vi "Dashboard Main_1366_768.vi"() -> ()   [LabVIEW 2020]
uses:
  <vilib>/event_ctls.llb/eventvkey.ctl
  <vilib>/Rock Robotics/WPI/Dashboard/WPI_DashboardLogging Global.vi
  <vilib>/Rock Robotics/Network Tables/NT Read Boolean.vi
panel:
  out "Camera Perf":string
  in  "Camera Settings":T1={"Frame Rate"=30, "Compression"=30, "Size"=1, "DB Camera Config"=FALSE} {"Frame Rate" scale=1.0..30.0; "Compression" scale=100.0..-1.0; "Size" items=["640x480", "320x240", "160x120"]}
  in  "TCP":refnum<k5>
  in  "Rec Mode":enum32{"Stop", "Record", "Playback"}(radio)
  out "Robot IP":string
  out "Image Message":string="Timeout in Camera Communications"
  in  "Dashboard Tab":T2(tab)
  in  "Select Auto":string(combo)="Select Autonomous ..."
  out "NT Connection":bool
  out "JS1 Z":dbl(slide) scale=-1.0..1.0 scale format="%#_2e"
  out "JS1 Graph":cluster{"X":dbl, "Y":dbl}[](graph)
  out "JS1 Buttons":T3
  out "JS2 Z":dbl(slide) scale=-1.0..1.0 scale format="%#_2e"
  out "JS2 Graph":cluster{"X":dbl, "Y":dbl}[](graph)
  out "JS2 Buttons":T3
  out "Mode":T4(ring)=enum."Auto Disabled"
  out "Right Camera Perf":cluster{"Bandwidth (Mbps)":dbl, "FPS":dbl}
  out "Middle":bool
  out "Bottom":bool
  out "Game\nPiece":bool
  out "Top":bool
  out "Shelf":bool
  out "Floor":bool
  out "MtT":bool
  out "At Target":bool
  out "Arm Override":bool
  out "Speed Modifer":dbl
  out "Reverse":bool
  out "Current Action":string
  out "ExtendDmd":dbl
  out "LiftDmd":dbl
  in  "DB/String 9":string
  in  "DB/String 8":string
  in  "DB/String 7":string
  in  "DB/String 6":string
  in  "DB/String 5":string
  in  "DB/String 4":string
  in  "DB/String 3":string
  in  "DB/String 2":string
  in  "DB/String 1":string
  in  "DB/String 0":string
  in  "DB/Slider 0":dbl(slide) scale=0.0..5.0
  in  "DB/Slider 1":dbl(slide) scale=0.0..5.0
  in  "DB/Slider 2":dbl(slide) scale=0.0..5.0
  in  "DB/Slider 3":dbl(slide) scale=0.0..5.0
  out "DB/LED 3":bool
  out "DB/LED 2":bool
  out "DB/LED 1":bool
  out "DB/LED 0":bool
  in  "DB/Button 3":bool
  in  "DB/Button 2":bool
  in  "DB/Button 1":bool
  in  "DB/Button 0":bool caption="New Name"
  in  "Test Slider":dbl(slide) scale=0.0..100.0 scale format="%#_3g"
  in  "On/Off":bool caption="Solenoid"
  in  "Test Name":u16(ring) items=["Select the test to run..."]
  in  "Test Tree":string(tree)
  in  "Motor":cluster{"Value":dbl, "Enable":bool} {"Value" scale=-1.0..1.0 scale format="%#_3g"}
  out "Progress":T5 {"Test Progress" scale=0.0..100.0}
  in  "Rev/Fwd":cluster{"Forward":bool, "Reverse":bool}
  in  "Test Ring":u16(ring) items=["Monochrome", "Color"]
  in  "CheckList":i32(listbox)
  out "Tree":string(tree)
  out "Camera Image":T6(plugin-control)
  out "Background":bool
  in  "Camera Name":string(combo)="No Camera Selection"
  # "HW"
  # "Joysticks"
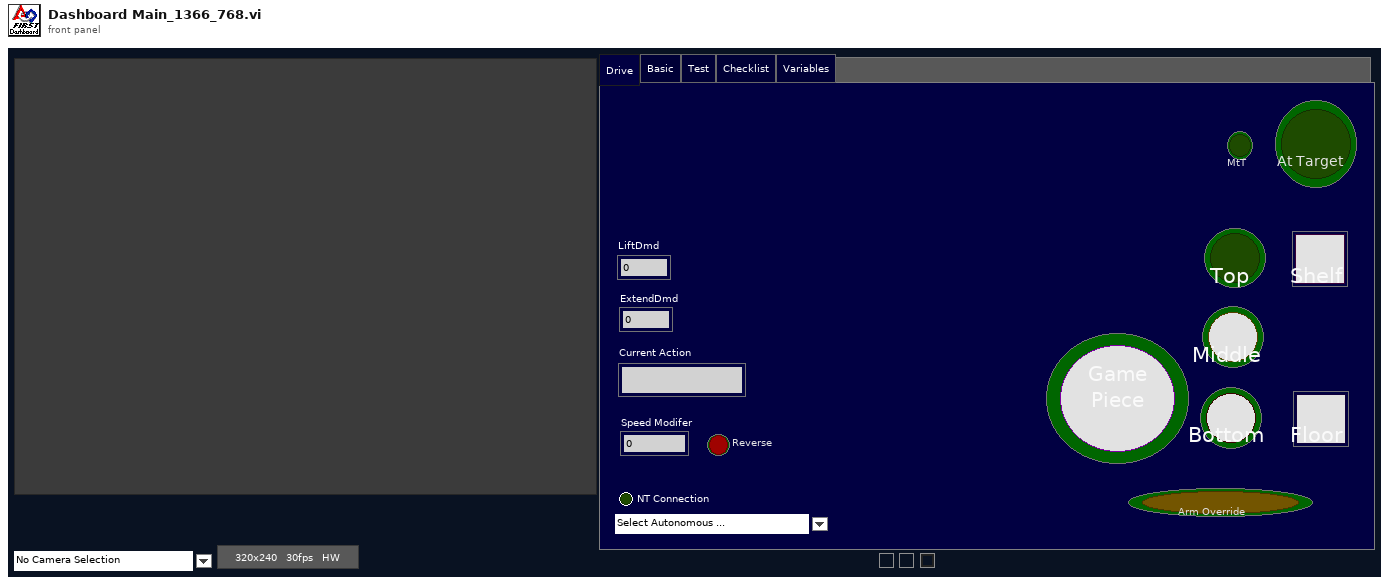
[diagram p1: front panel]
types:
  T1 = cluster{"Frame Rate":i32, "Compression":i32, "Size":u16, "DB Camera Config":bool}
  T2 = enum32{"Drive", "Basic", "Test", "Checklist", "Variables"}
  T3 = cluster{bool, bool, bool, bool, bool, bool, bool, bool, bool, bool, bool, bool}
  T4 = enum8{"Tele-Op Disabled", "Tele-Op Enabled", "Auto Disabled", "Auto Enabled", "Test Disabled", "Test Enabled", "Disconnected", "No Code", "E-Stop"}
  T5 = cluster{"Test Progress":u8, "Test Progress Text":string}
  T6 = typedef "IMAQ Image.ctl" = refnum<image>
  T7 = enum32{"Drive", "Basic", "Custom", "Test", "Checklist", "Variables"}
  T8 = cluster{"Save Path":path, "Interval (s)":dbl, "Keep":i32}
  T9 = enum32{"Drive", "Camera", "Basic", "Custom", "Test", "Commands", "Checklist", "Variables"}
  T10 = typedef "Image Type" = u32
  T11 = cluster{"Error Strings":string, "Disable Counts":cluster{u16, u16}, "Rail Faults":cluster{u16, u16, u16}, "Robot IP":string, "DB Mode":u8, "Event Info":cluster{"Name":string, "Type":u8, "Number":u16, "Replay":u8}}
  T12 = cluster{"Storage":cluster{"Disk Free":u64, "RAM Block":u32, "RAM free":u32}, "CPU Utilization":cluster{"CPU % ISR":sgl, "CPU % Time Crit":sgl, "CPU % Timed Str":sgl, "CPU % High":sgl, "CPU % Above":sgl, "CPU % Normal":sgl, "CPU % Low":sgl}, "CAN":cluster{"% Bus Utilization":sgl, "Bus Off Cnt":u32, "TX_FIFO Full Cnt":u32, "Receive Error Cnt":u8, "Transmit Error Cnt":u8}, "HID":cluster{"HID Outputs":u32, "Rumble Low":u16, "Rumble High":u16}[]}
  T13 = cluster{"Status bits":cluster{"Test Mode":bool, "Autonomous":bool, "Enabled":bool, "Code Start":bool, "Brownout":bool, "Reserved 2":bool, "Reserved 3":bool, "E-Stop":bool}, "Code Trace":cluster{"Disabled":bool, "TeleOp":bool, "Auto":bool, "Test":bool}, "Controller Type":enum16{"unknown", "cRIO", "roboRio"}, "Code?":enum16{"unknown", "noCode", "code"}, "Battery V":dbl}
  T14 = cluster{"Control Bits":cluster{"TestMode":bool, "Autonomous":bool, "Enabled":bool, "FMS Present":bool, bool, bool, bool, "E-Stop":bool}, "Team Station ":u8, "Countdown":sgl, "Joystick Values":cluster{"Axes":dbl[], "Buttons":bool[], "POVs":i16[]}[]}
  T15 = cluster{"Axes":dbl[], "Buttons":bool[], "POVs":i16[]}[]
  T16 = cluster{"Axes":dbl[], "Buttons":bool[], "POVs":i16[]}
  T17 = cluster{"Buttons[0]":bool, "Buttons[1]":bool, "Buttons[2]":bool, "Buttons[3]":bool, "Buttons[4]":bool, "Buttons[5]":bool, "Buttons[6]":bool, "Buttons[7]":bool, "Buttons[8]":bool, "Buttons[9]":bool, "Buttons[10]":bool, "Buttons[11]":bool}
  T18 = cluster{"Camera Image":refnum<vi>, "Dashboard Tab":refnum<vi>, "Background":refnum<vi>, "Rec Mode":refnum<vi>, "Test Slider":refnum<vi>, "On/Off ":refnum<vi>, "Test Ring":refnum<vi>, "Rev/Fwd":refnum<vi>, "Test Name":refnum<vi>, "Motor":refnum<vi>, "Progress":refnum<vi>, "CheckList":refnum<vi>, "Tree":refnum<vi>, "Test Tree":refnum<vi>, "Camera Settings":refnum<vi>, "Camera Name":refnum<vi>, "Camera Perf":refnum<vi>}
  T19 = cluster{"Global Rectangle":i32[], "Contours":cluster{"Contour Type":u32, "ROI Type":u32, "Points":i32[]}[]}
  T20 = cluster{"Camera Name":string, string, "Saved DB Images Info":cluster{"Save Path":path, "Interval (s)":dbl, "Keep":i32}}
  T21 = cluster{"Operation":enum16{"Update", "Clear"}, "Color Box":u32}[]
  T22 = typedef "eventvkey.ctl" = enum16{"ASCII", "Enter", "Return", "Shift", "Ctrl", "Alt", "Cmd", "Opt", "Caps", "NumLock", "Clear", "Break", "Up", "Down", "Left", "Right", "Insert", "Delete", "Home", "End", "PageUp", "PageDown", "Escape", "Help", "Pause", "ScrollLock", "F1", "F2", "F3", "F4", "F5", "F6", "F7", "F8", "F9", "F10", "F11", "F12", "F13", "F14", "F15", "F16", "F17", "F18", "F19", "F20", "F21", "F22", "F23", "F24", "Play", "VolumeUp", "VolumeDown", "Mute", "Two Byte Char"}
  T23 = cluster{"Image Size":bool, "Image Type":bool, "Pixel Value":bool, "ROI Information":bool, "Zoom Factor":bool}
  T24 = cluster{"Operation":enum16{"Update", "Clear"}, "Color Box":u32}
  T25 = cluster{"Shift":bool, "Ctrl":bool, "Alt":bool, "Cmd":bool, "Opt":bool}
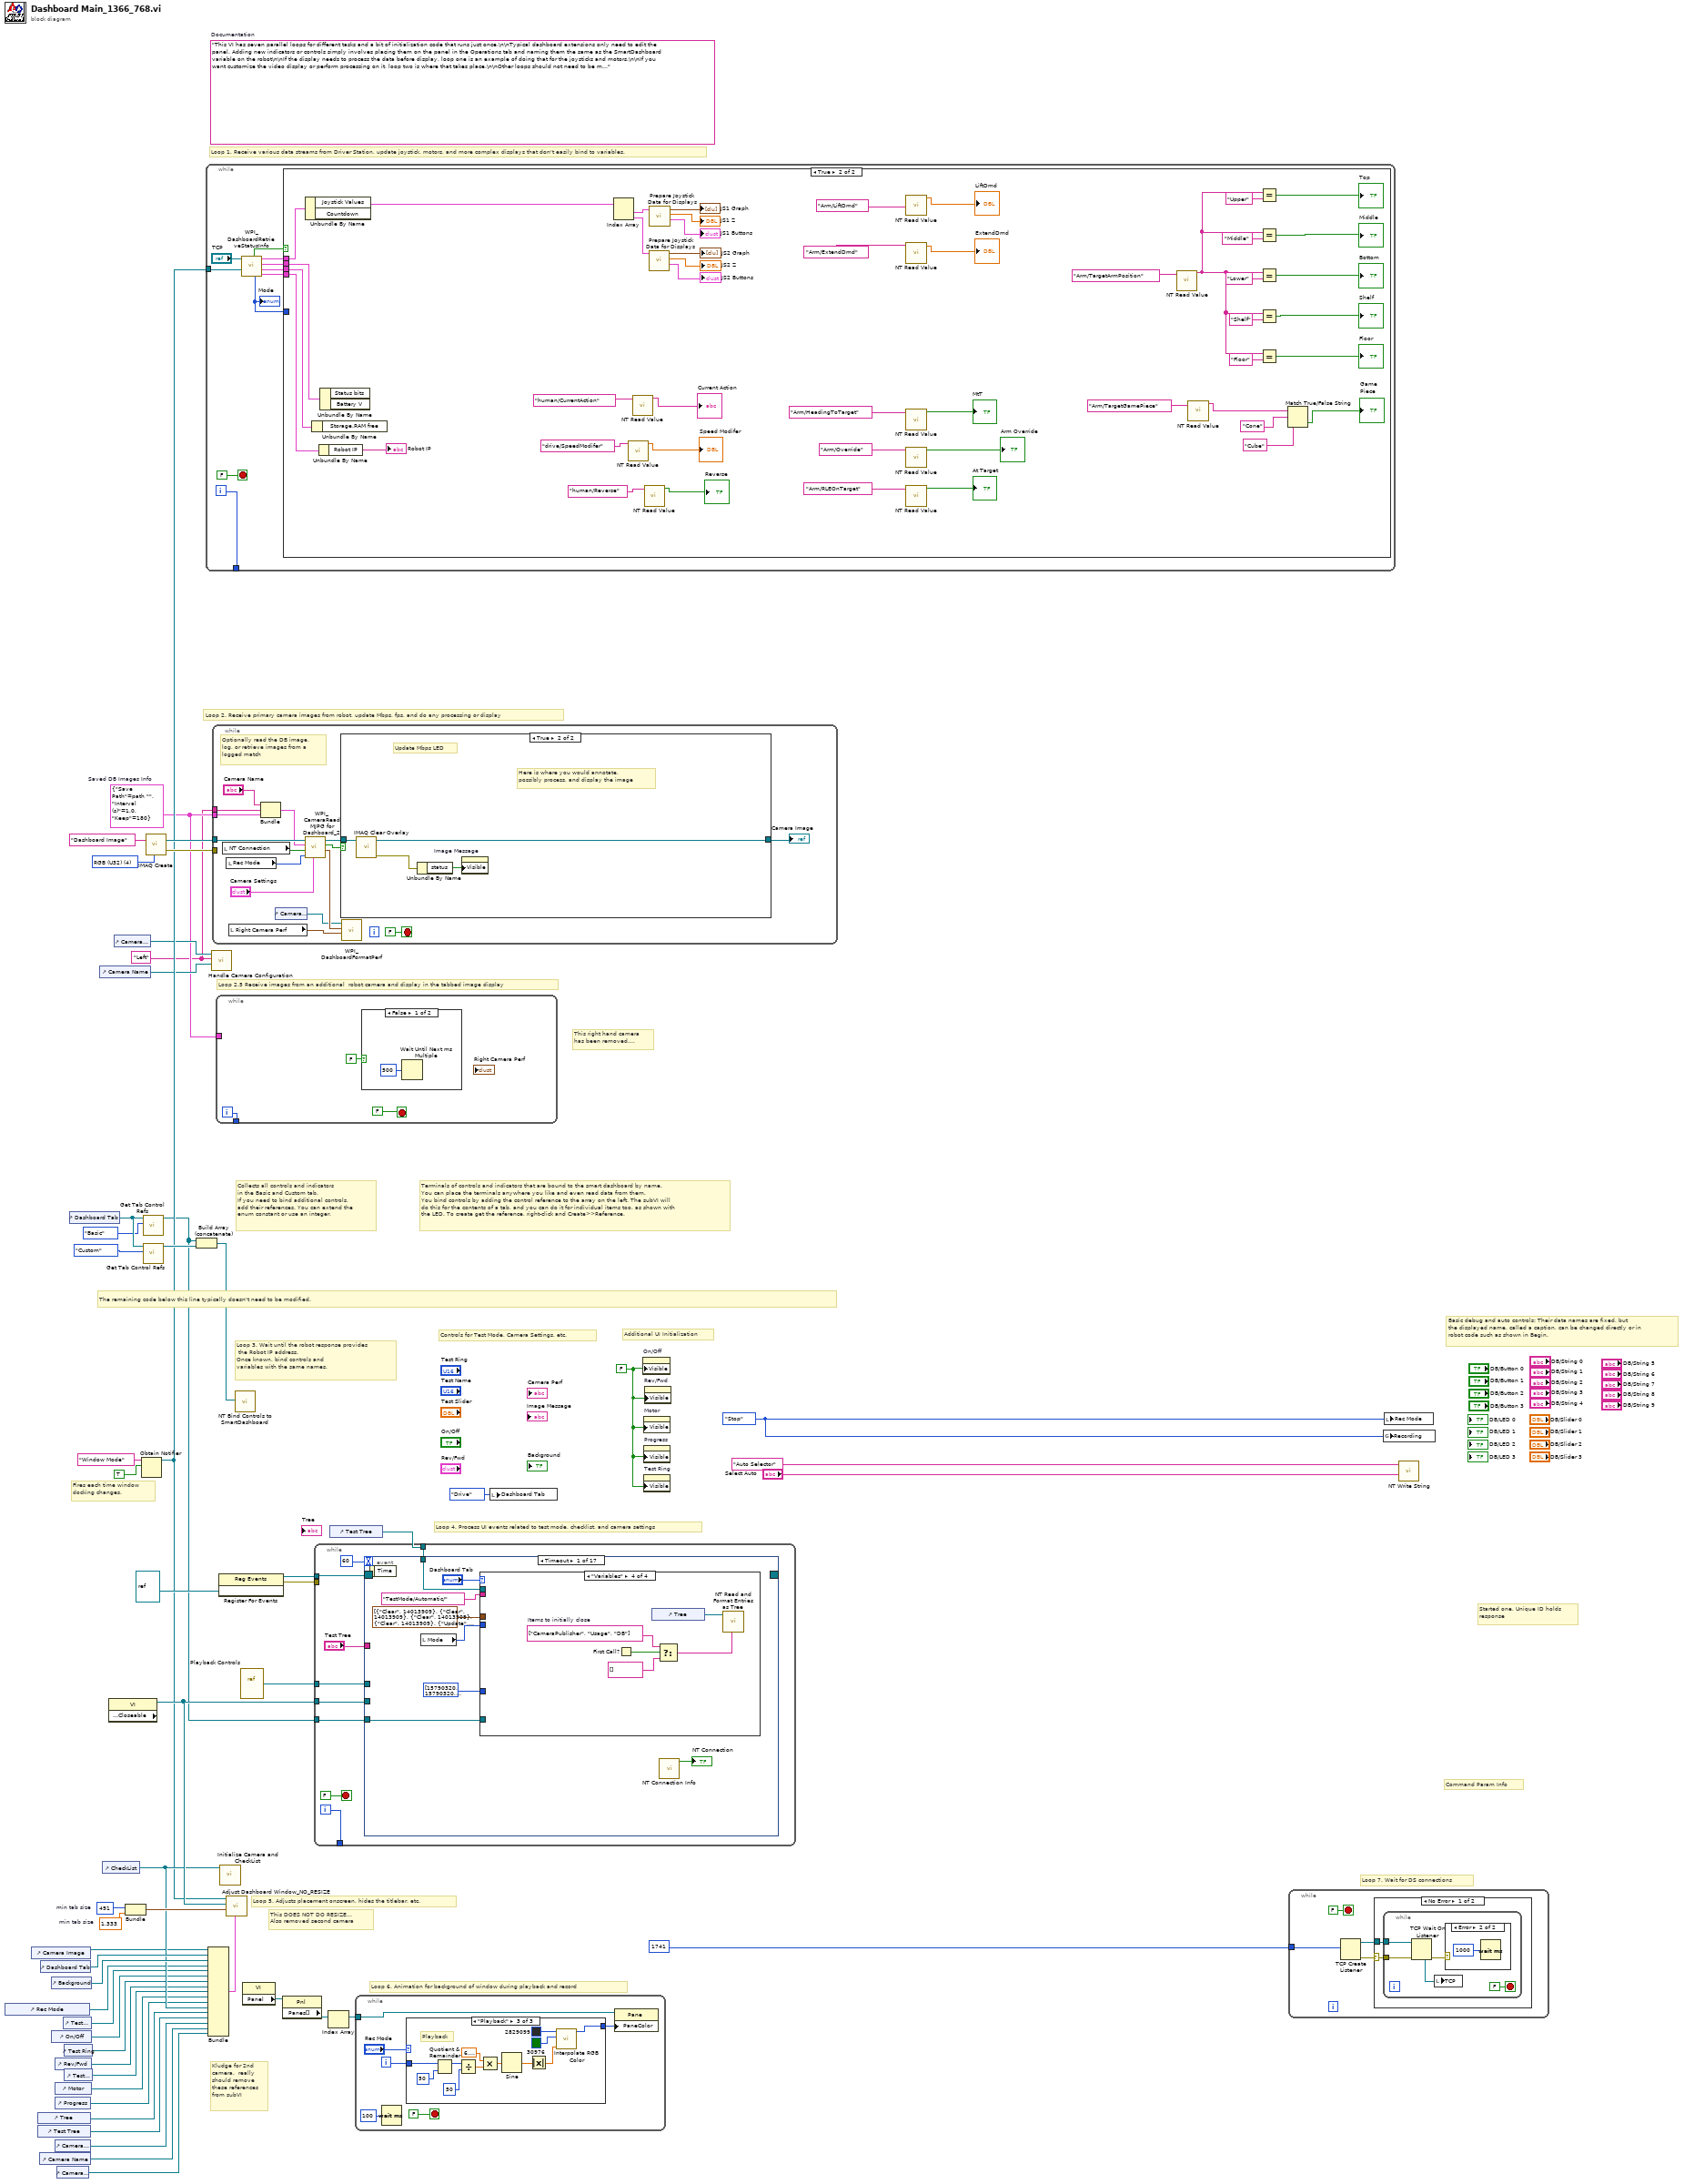
[diagram p0: block diagram]
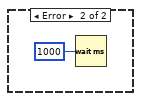
[diagram p4: hidden frame]
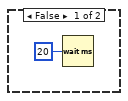
[diagram p5: hidden frame]
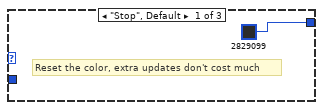
[diagram p6: hidden frame]
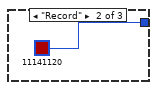
[diagram p7: hidden frame]
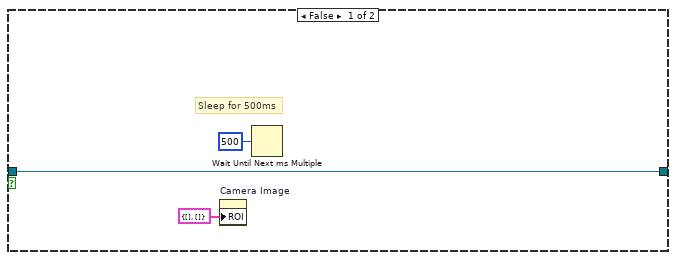
[diagram p8: hidden frame]
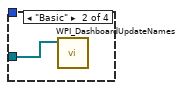
[diagram p10: hidden frame]
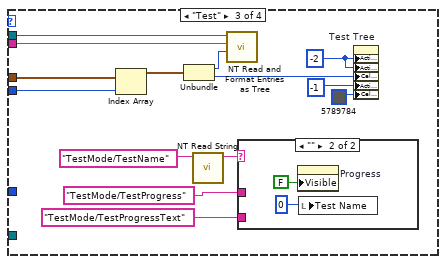
[diagram p11: hidden frame]
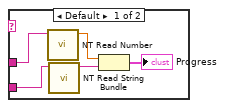
[diagram p12: hidden frame]
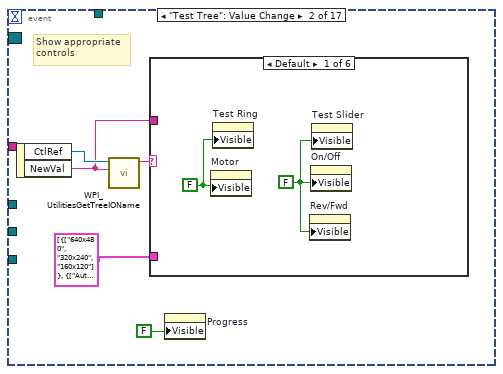
[diagram p13: hidden frame]
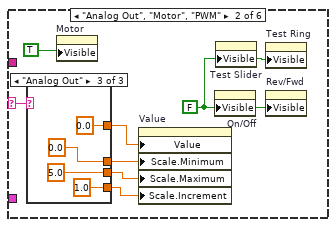
[diagram p14: hidden frame]
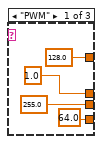
[diagram p15: hidden frame]
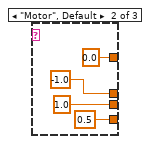
[diagram p16: hidden frame]
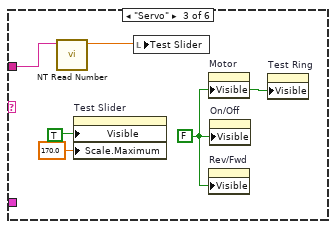
[diagram p17: hidden frame]
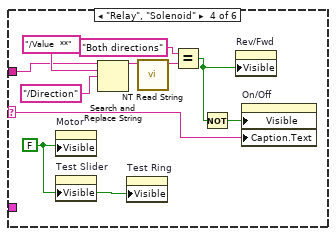
[diagram p18: hidden frame]
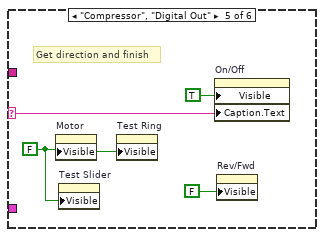
[diagram p19: hidden frame]
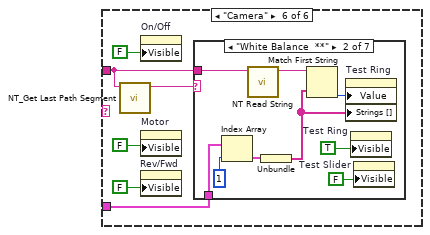
[diagram p20: hidden frame]
diagram:
  w6 = T8 {"Save Path"=path "", "Interval (s)"=1.0, "Keep"=180}  # Saved DB Images Info
  w5 = "Left"
  w33 = 491  # min tab size
  w32 = 1.333  # min tab size
  w39 = enum32{"Stop", "Record", "Playback"}."Stop" ("Rec Mode")
  w17 = FALSE ("Visible")
  (unwired) "This VI has seven parallel loops for different tasks and a bit of initialization code that runs just once.\n\nTypical dashboard extensions only need to edit the panel. Adding new indicators or controls simply involves placing them on the panel in the Operations tab and naming them the same as the SmartDashboard variable on the robot\n\nIf the display needs to process the data before display, loop one is an example of doing that for the joysticks and motors.\n\nIf you want customize the video display or perform processing on it, loop two is where that takes place.\n\nOther loops should not need to be modified. They are pretty standard, and document the task they perform."  # Documentation
  w53 = T10 4 items=["Grayscale (U8)", "Grayscale (I16)", "Grayscale (SGL)", "Complex (CSG)", "RGB (U32)", "HSL (U32)", "RGB (U64)"] ("Image Type")
  # "Kludge for 2nd\ncamera.  really\nshould remove\nthese references\nfrom subVI"
  # "This right hand camera\nhas been removed...."
  # "This DOES NOT DO RESIZE...\nAlso removed second camera"
  # "Loop 2.5 Receive images from an additional  robot camera and display in the tabbed image display"
  # "Command Param Info"
  # "Started one, Unique ID holds\nresponse"
  # "Loop 7. Wait for DS connections"
  # "Basic debug and auto controls: Their data names are fixed, but\nthe displayed name, called a caption, can be changed directly or in\nrobot code such as shown in Begin."
  # "Controls for Test Mode, Camera Settings, etc."
  # "Additional UI Initialization"
  # "Loop 6. Animation for background of window during playback and record"
  # "Fires each time window\ndocking changes."
  # "Collects all controls and indicators\nin the Basic and Custom tab.\nIf you need to bind additional controls,\nadd their references. You can extend the\nenum constant or use an integer."
  # "The remaining code below this line typically doesn't need to be modified."
  # "Loop 4. Process UI events related to test mode, checklist, and camera settings"
  # "Terminals of controls and indicators that are bound to the smart dashboard by name.\nYou can place the terminals anywhere you like and even read data from them.\nYou bind controls by adding the control reference to the array on the left. The subVI will\ndo this for the contents of a tab, and you can do it for individual items too, as shown with\nthe LED. To create get the reference, right-click and Create>>Reference."
  # "Loop 3. Wait until the robot response provides\n the Robot IP address.\nOnce known, bind controls and\nvariables with the same names."
  # "Loop 5. Adjusts placement onscreen, hides the titlebar, etc."
  # "Loop 1. Receive various data streams from Driver Station, update joystick, motors, and more complex displays that don't easily bind to variables."
  # "Loop 2. Receive primary camera images from robot, update Mbps, fps, and do any processing or display"
  n1 = control-ref of="Rec Mode"() -> (w23:refnum<vi>)
  n2 = control-ref of="Camera Image"() -> (w2:refnum<vi>)
  n3 = control-ref of="Tree"() -> (w27:refnum<vi>)
  n4 = control-ref of="Test Tree"() -> (w26:refnum<vi>)
  n5 = control-ref of="Camera Name"() -> (w3:refnum<vi>)
  n6 = control-ref of="Dashboard Tab"() -> (w34:refnum<vi>)
  n7 = control-ref of="Background"() -> (w30:refnum<vi>)
  n8 = control-ref of="On/Off"() -> (w21:refnum<vi>)
  n9 = control-ref of="Progress"() -> (w18:refnum<vi>)
  n10 = control-ref of="Camera Settings"() -> (w4:refnum<vi>)
  n11 = control-ref of="Rev/Fwd"() -> (w19:refnum<vi>)
  n12 = control-ref of="Motor"() -> (w24:refnum<vi>)
  n13 = control-ref of="Camera Perf"() -> (w12:refnum<vi>)
  n14 = control-ref of="Test Slider"() -> (w22:refnum<vi>)
  n15 = control-ref of="Test Ring"() -> (w20:refnum<vi>)
  n16 = control-ref of="Test Name"() -> (w25:refnum<vi>)
  n17 = control-ref of="Dashboard Tab"() -> (w37:refnum<vi>)
  n18 = control-ref of="Camera Name"() -> (w13:refnum<vi>)
  n19 = control-ref of="CheckList"() -> (w28:refnum<vi>)
  n20 = property class="VI" props=["Front Panel.Closeable"]() -> (reference out=w38:refnum<vi>)  [unwired: 2 in, 2 out]
  n21 = control-ref of="Camera Settings"() -> (w14:refnum<vi>)
  n22 = Bundle("min tab size"=w33, "min tab size"=w32) -> (w31:cluster{"min tab size":i32, "min tab size":dbl})  [unwired: 1 in]
  n23 = Obtain Notifier(name (unnamed)="Window Mode", notification data type=TRUE) -> (notifier out=w16:refnum<notifier>)  [unwired: 2 in, 2 out]
  n24 = call <vilib>:"Get Tab Control Refs.vi"("Page Index"=T9."Basic" ("Dashboard Tab"), "TabControl in"=w37) -> ("ControlsOnPage"=w11:refnum<vi>[])  [unwired: 9 in]
  n25 = call <vilib>:"Get Tab Control Refs.vi"("Page Index"=T9."Custom" ("Dashboard Tab"), "TabControl in"=w37) -> ("ControlsOnPage"=w36:refnum<vi>[])  [unwired: 9 in]
  n26 = call "IMAQ Create"("Image Name"="Dashboard Image", "Image Type"=w53) -> ("New Image"=w51:T6, "error out"=w50:errorcluster)  [unwired: 2 in, 1 out]
  n27 = Build Array (concatenate)(w11, w36) -> (w35:refnum<vi>[])
  n28 = while {
    tunnel: [w62] -> _
    tunnel: w16 -> [w54]
    i -> [w62]
    stop <- FALSE stop-if-true
    n29 = call <vilib>:"WPI_DashboardRetrieveStatusInfo.vi"("Window Mode Notifier"=w54, "TCP Cnx"="TCP") -> ("Power and Errors"=w57:T11, "Robot Metrics"=w60:T12, "Status Info"=w61:T13, "Control Info"=w58:T14, "Robot Mode"=w56:T4, "Process?"=w59:bool)  [unwired: 4 in]
    "Mode" <- w56
    n30 = case shown="True" w59 {
      tunnel: w61 -> [_ w111]
      tunnel: w60 -> [_ w110]
      tunnel: w58 -> [_ w109]
      tunnel: w57 -> [_ w108]
      tunnel: w56 -> [_ _]
      frame False {
        n31 = Wait (ms)(milliseconds to wait=u32 20) -> ()  [unwired: 1 out]
      }
      frame True {
        n32 = Unbundle By Name(w109) -> ("Joystick Values"=w107:T15)  [unwired: 1 out]
        n33 = Unbundle By Name(w110) -> ()  [unwired: 1 out]
        n34 = Unbundle By Name(w108) -> ("Robot IP"=→"Robot IP":string)
        n35 = Unbundle By Name(w111) -> ()  [unwired: 2 out]
        n36 = Index Array(array=w107) -> (element #1=w106:T16, element #2=w102:T16)  [unwired: 2 in]
        n37 = call-poly <vilib>:"NT Read Value.vi"("name"="drive/SpeedModifer") -> ("value"=→"Speed Modifer":dbl)  [unwired: 8 in, 2 out]
        n38 = call-poly <vilib>:"NT Read Value.vi"("name"="human/CurrentAction") -> ("value"=→"Current Action":string)  [unwired: 8 in, 2 out]
        n39 = call-poly <vilib>:"NT Read Value.vi"("name"="human/Reverse") -> ("value"=→"Reverse":bool)  [unwired: 8 in, 2 out]
        n40 = call "Prepare Joystick Data for Displays.vi"("Joystick Values"=w102) -> ("Buttons"=→"JS2 Buttons":T17, "Z Axis"=→"JS2 Z":dbl, "Cartesian Data"=→"JS2 Graph":cluster{"X axis":dbl, "X axis":dbl}[])  [unwired: 8 in]
        n41 = call "Prepare Joystick Data for Displays.vi"("Joystick Values"=w106) -> ("Buttons"=→"JS1 Buttons":T17, "Z Axis"=→"JS1 Z":dbl, "Cartesian Data"=→"JS1 Graph":cluster{"X axis":dbl, "X axis":dbl}[])  [unwired: 8 in]
        n42 = call-poly <vilib>:"NT Read Value.vi"("name"="Arm/LiftDmd") -> ("value"=→"LiftDmd":dbl)  [unwired: 8 in, 2 out]
        n43 = call-poly <vilib>:"NT Read Value.vi"("name"="Arm/ExtendDmd") -> ("value"=→"ExtendDmd":dbl)  [unwired: 8 in, 2 out]
        n44 = call-poly <vilib>:"NT Read Value.vi"("name"="Arm/HeadingToTarget") -> ("value"=→"MtT":bool)  [unwired: 8 in, 2 out]
        n45 = call-poly <vilib>:"NT Read Value.vi"("name"="Arm/Override") -> ("value"=→"Arm Override":bool)  [unwired: 8 in, 2 out]
        n46 = call-poly <vilib>:"NT Read Value.vi"("name"="Arm/RLEOnTarget") -> ("value"=→"At Target":bool)  [unwired: 8 in, 2 out]
        n47 = call-poly <vilib>:"NT Read Value.vi"("name"="Arm/TargetArmPosition") -> ("value"=w80:string)  [unwired: 8 in, 2 out]
        n48 = call-poly <vilib>:"NT Read Value.vi"("name"="Arm/TargetGamePiece") -> ("value"=w73:string)  [unwired: 8 in, 2 out]
        n49 = Equal?(x=w80, y="Upper") -> (x = y?=→"Top":bool)
        n50 = Equal?(x=w80, y="Middle") -> (x = y?=→"Middle":bool)
        n51 = Equal?(x=w80, y="Lower") -> (x = y?=→"Bottom":bool)
        n52 = Equal?(x=w80, y="Shelf") -> (x = y?=→"Shelf":bool)
        n53 = Equal?(x=w80, y="Floor") -> (x = y?=→"Floor":bool)
        n54 = Match True/False String(2:"Cube" ("false string"), 3:"Cone" ("true string"), 4:w73) -> (0:→"Game\nPiece":bool)  [unwired: 1 out]
      }
    }
  }
  n55 = Bundle("Camera Image"=w2, "Dashboard Tab"=w34, "Background"=w30, "Rec Mode"=w23, "Test Slider"=w22, "On/Off"=w21, "Test Ring"=w20, "Rev/Fwd"=w19, "Test Name"=w25, "Motor"=w24, "Progress"=w18, "CheckList"=w28, "Tree"=w27, "Test Tree"=w26, "Camera Settings"=w4, "Camera Name"=w3, "Camera Perf"=w12) -> (w29:T18)  [unwired: 1 in]
  n56 = call "Handle Camera Configuration.vi"("CameraNameRef"=w13, "Display Name"=w5, "ClusterRef"=w14) -> ()  [unwired: 9 in]
  n57 = while {
    tunnel: w51 -> [w125]
    tunnel: w50 -> [_]
    tunnel: w6 -> [w118]
    tunnel: w5 -> [w115]
    stop <- FALSE stop-if-true
    # "Optionally read the DB image,\nlog, or retrieve images from a\nlogged match"
    n58 = local read "NT Connection"() -> (w119:bool)
    n59 = local read "Rec Mode"() -> (w122:enum32{"Stop", "Record", "Playback"})
    n60 = local read "Right Camera Perf"() -> (w113:cluster{"Bandwidth (Mbps)":dbl, "FPS":dbl})
    n61 = Bundle("Camera Name"="Camera Name", w115, "Saved DB Images Info"=w118) -> (w117:T20)  [unwired: 1 in]
    n62 = control-ref of="Camera Perf"() -> (w112:refnum<vi>)
    n63 = call <vilib>:"WPI_CameraRead MJPG for Dashboard_2.vi"("Camera Settings"="Camera Settings", "Rec Mode"=w122, "NT Connection"=w119, "Capture Info"=w117, "Image in"=w125) -> ("perf info"=w114:cluster{"Bandwidth (Mbps)":dbl, "fps":dbl}, "Active"=w123:bool, "Image\\ out"=w124:T6)  [unwired: 4 in]
    n64 = case shown="True" w123 {
      tunnel: w124 -> [w128 w131]
      tunnel: [w128 w130] -> w120
      frame False {
        # "Sleep for 500ms"
        n65 = property on="Camera Image" class="ImageControl"("ROI"=T19 {"Global Rectangle"=[], "Contours"=[]}) -> ()  [unwired: 2 in, 2 out]
        n66 = Wait Until Next ms Multiple(millisecond multiple=u32 500) -> ()  [unwired: 1 out]
      }
      frame True {
        # "Here is where you would annotate,\npossibly process, and display the image"
        # "Update Mbps LED"
        n67 = call "IMAQ Clear Overlay"("Image"=w131) -> ("error out"=w132:errorcluster, "Image Out"=w130:T6)  [unwired: 2 in, 7 out]
        n68 = Unbundle By Name(w132) -> ("status"=w133:bool)
        n69 = property on="Image Message" class="Str"("Visible"=w133) -> ()  [unwired: 2 in, 2 out]
      }
    }
    "Camera Image" <- w120
    n70 = call <vilib>:"WPI_DashboardFormatPerf.vi"("Right Camera Perf"=w113, "Performance"=w114, "String in"=w112) -> ()  [unwired: 9 in]
  }
  n71 = while {
    tunnel: [w135] -> _
    tunnel: w6 -> [_]
    i -> [w135]
    stop <- FALSE stop-if-true
    n72 = case shown="False" FALSE {
      frame False {
        n73 = Wait Until Next ms Multiple(millisecond multiple=u32 500) -> ()  [unwired: 1 out]
      }
      frame True {
      }
    }
  }
  n74 = register-events(refnum<vi> refnum) -> (reference out=w42:refnum<event-registration>, error out=w41:errorcluster)  [unwired: 2 in]
  n75 = call "Initialize Camera and CheckList.vi"("ListBox in"=w28) -> ()  [unwired: 11 in]
  n76 = call "Adjust Dashboard Window_NO_RESIZE.vi"("Sizing Refnums"=w29, "Size Constraints"=w31, "VI"=w38, "WIn Mode"=w16) -> ()  [unwired: 8 in]
  n77 = call <vilib>:"NT Bind Controls to SmartDashboard.vi"("Bound Control Refs"=w35) -> ()  [unwired: 11 in]
  n78 = vi-ref "Playback Controls.vi"() -> (w43:refnum<vi>)
  n79 = property class="VI"() -> ("Panel"=w45:refnum<vi>)  [unwired: 2 in, 2 out]
  n80 = property class="Pnl"(reference=w45) -> ("Panes[]"=w46:refnum<vi>[])  [unwired: 1 in, 2 out]
  n81 = Index Array(array=w46) -> (element=w44:refnum<vi>)  [unwired: 1 in]
  n82 = control-ref of="Test Tree"() -> (w47:refnum<vi>)
  n83 = while {
    tunnel: [w143] -> _
    tunnel: w47 -> [w142]
    tunnel: w43 -> [w141]
    tunnel: w42 -> [w140]
    tunnel: w41 -> [_]
    tunnel: w38 -> [w139]
    tunnel: w11 -> [w138]
    i -> [w143]
    stop <- FALSE stop-if-true
    n84 = event shown="[0] Timeout" {
      selector: w140 -> [_ _ _ _ _ _ _ _ _ _ _ _ _ _ _ _ _]
      dyn-events: [_ _ _ _ _ _ _ _ _ _ _ _ _ w348 _ _ _] -> _
      timeout: u32 60 ("milliseconds to wait") -> [_ _ _ _ _ _ _ _ _ _ _ _ _ _ _ _ _]
      tunnel: w142 -> [w153 _ _ _ _ _ _ _ _ _ _ _ _ _ _ _ _]
      tunnel: "Test Tree" -> [_ _ _ _ _ _ _ _ w321 w328 w329 w332 w339 _ _ _ _]
      tunnel: w141 -> [_ _ _ _ _ _ _ _ _ _ _ _ _ w350 _ w365 _]
      tunnel: w139 -> [_ _ _ _ _ _ _ _ _ _ _ _ _ w346 _ _ _]
      tunnel: w138 -> [w148 _ _ _ _ _ _ _ _ _ _ _ _ _ _ _ _]
      event Timeout {
        n85 = event-data() -> ()  [unwired: 1 in, 1 out]
        n86 = local read "Mode"() -> (w151:T4)
        n87 = case shown="\"Variables\"" "Dashboard Tab" {
          tunnel: w153 -> [_ _ w169 _]
          tunnel: "TestMode/Automatic/" ("Name Pattern") -> [_ _ w168 _]
          tunnel: T21 [{"Operation"=enum."Clear", "Color Box"=14013909}, {"Operation"=enum."Clear", "Color Box"=14013909}, {"Operation"=enum."Clear", "Color Box"=14013909}, {"Operation"=enum."Clear", "Color Box"=14013909}, {"Operation"=enum."Update", "Color Box"=14013909}, {"Operation"=enum."Update", "Color Box"=16777215}, {"Operation"=enum."Clear", "Color Box"=14013909}, {"Operation"=enum."Clear", "Color Box"=14013909}, {"Operation"=enum."Clear", "Color Box"=14013909}] -> [_ _ w161 _]
          tunnel: w151 -> [_ _ w160 _]
          tunnel: u32[] [15790320, 15790320, 15790320, 15790320, 16777215, 16777215, 15790320, 15790320, 15790320] -> [_ _ _ _]
          tunnel: w148 -> [_ w155 _ _]
          frame "Test", Default {
          }
          frame "Basic" {
            n88 = call <vilib>:"WPI_DashboardUpdateNames.vi"("Controls on Tab"=w155) -> ()  [unwired: 11 in]
          }
          frame "Test" {
            w167 = -2 ("Active Item:Row Number")
            n89 = Index Array(array=w161, index=w160) -> (element=w162:T24)
            n90 = Unbundle(w162) -> ("Operation"=w163:enum16{"Update", "Clear"}, "Color Box"=w164:u32)
            n91 = call <vilib>:"NT Read String.vi"("name"="TestMode/TestName" ("Name")) -> ("value"=w158:string)  [unwired: 8 in, 2 out]
            n92 = call <vilib>:"NT Read and Format Entries as Tree.vi"("Operation"=w163, "Name Pattern"=w168, "Tree Refnum"=w169) -> ()  [unwired: 7 in, 2 out]
            n93 = case shown="\"\"" w158 {
              tunnel: "TestMode/TestProgress" ("Name") -> [w171 _]
              tunnel: "TestMode/TestProgressText" ("Name") -> [w170 _]
              frame Default {
                n94 = call <vilib>:"NT Read Number.vi"("name"=w171) -> ("value"=w172:dbl)  [unwired: 8 in, 2 out]
                n95 = call <vilib>:"NT Read String.vi"("name"=w170) -> ("value"=w173:string)  [unwired: 8 in, 2 out]
                n96 = Bundle("value"=w172, "value"=w173) -> (→"Progress":cluster{"value":dbl, "value":string})  [unwired: 1 in]
              }
              frame "" {
                n97 = property on="Progress" class="Clust (strict)"("Visible"=FALSE) -> ()  [unwired: 2 in, 2 out]
                n98 = local write "Test Name"(u16 0) -> ()
              }
            }
            n99 = property on="Test Tree" class="Tree (strict)"("Active Item Row Number"=w167, "ActiveColNum"=w167, "CellBG"=w164, "Active Item Row Number"=-1 ("Active Item:Row Number"), "CellBG"=u32 5789784 ("Color Box")) -> ()  [unwired: 2 in, 2 out]
          }
          frame "Variables" {
            w179 = string[] ["CameraPublisher", "Usage", "DB"]  # Items to initially close
            n100 = First Call?() -> (First Call?: T/F=w180:bool)
            n101 = control-ref of="Tree"() -> (w181:refnum<vi>)
            n102 = Select(t=w179, s=w180, f=string[] []) -> (s? t:f=w177:string[])
            n103 = call <vilib>:"NT Read and Format Entries as Tree.vi"("Tags to  Close"=w177, "Tree Refnum"=w181) -> ()  [unwired: 8 in, 2 out]
          }
        }
        n104 = call <vilib>:"NT Connection Info.vi"() -> ("Connected"=→"NT Connection":bool)  [unwired: 11 in]
      }
      event "Test Tree": Value Change {
        # "Show appropriate\ncontrols"
        n105 = event-data() -> ("CtlRef"=w185:refnum<vi>, "NewVal"=w183:string)  [unwired: 1 in]
        n106 = call <vilib>:"WPI_UtilitiesGetTreeIOName.vi"("NewVal"=w183, "TreeControl in"=w185) -> ("I/O Name"=w186:string)  [unwired: 9 in]
        n107 = case shown="Default" w186 {
          selector: w186 -> [_ w193 _ w215 w224 _]
          tunnel: w183 -> [_ _ w212 w214 _ w231]
          tunnel: cluster{string[]}[] [{["640x480", "320x240", "160x120"]}, {["Auto", "Fixed indoor", "Fixed outdoor 1", "Fixed outdoor 2", "Fixed fluorescent 1", "Fixed fluorescent 2", "Hold current"]}, {["Auto", "Flicker-free 50 Hz", "Flicker-free 60 Hz", "Hold current"]}, {["None", "Prioritize frame rate", "Prioritize image quality"]}, {["Monochrome", "Color"]}] -> [_ _ _ _ _ w230]
          frame Default {
            w188 = FALSE ("Visible")
            w187 = FALSE ("Visible")
            n108 = property on="Motor" class="Clust (strict)"("Visible"=w187) -> ()  [unwired: 2 in, 2 out]
            n109 = property on="Test Ring" class="Ring (strict)"("Visible"=w187) -> ()  [unwired: 2 in, 2 out]
            n110 = property on="Rev/Fwd" class="Clust (strict)"("Visible"=w188) -> ()  [unwired: 2 in, 2 out]
            n111 = property on="On/Off" class="Bool (strict)"("Visible"=w188) -> ()  [unwired: 2 in, 2 out]
            n112 = property on="Test Slider" class="Slide (strict)"("Visible"=w188) -> ()  [unwired: 2 in, 2 out]
          }
          frame "Analog Out", "Motor", "PWM" {
            w194 = FALSE ("Visible")
            n113 = case shown="\"Analog Out\"" w193 {
              tunnel: [1.0 ("Value") -1.0 ("Value") 0.0 ("Value")] -> w192
              tunnel: [255.0 ("Value") 1.0 ("Value") 5.0 ("Value")] -> w191
              tunnel: [128.0 ("Value") 0.0 ("Value") 0.0 ("Value")] -> w190
              tunnel: [64.0 ("Value") 0.5 ("Value") 1.0 ("Value")] -> w189
              frame "PWM" {
              }
              frame "Motor", Default {
              }
              frame "Analog Out" {
              }
            }
            n114 = property on="Motor" class="Clust (strict)"("Visible"=TRUE) -> ()  [unwired: 2 in, 2 out]
            n115 = property on="Value" class="Slide (strict)"("Value"=w190, "Scale.Minimum"=w192, "Scale.Maximum"=w191, "Scale.Increment"=w189) -> ()  [unwired: 2 in, 2 out]
            n116 = property on="On/Off" class="Bool (strict)"("Visible"=w194) -> ()  [unwired: 2 in, 2 out]
            n117 = property on="Test Slider" class="Slide (strict)"("Visible"=w194) -> ()  [unwired: 2 in, 2 out]
            n118 = property on="Test Ring" class="Ring (strict)"("Visible"=w194) -> ()  [unwired: 2 in, 2 out]
            n119 = property on="Rev/Fwd" class="Clust (strict)"("Visible"=w194) -> ()  [unwired: 2 in, 2 out]
          }
          frame "Servo" {
            w210 = FALSE ("Visible")
            n120 = call <vilib>:"NT Read Number.vi"("name"=w212) -> ("value"=w211:dbl)  [unwired: 8 in, 2 out]
            n121 = property on="Test Slider" class="Slide (strict)"("Visible"=TRUE, "Scale.Maximum"=170.0 ("Scale.Range:Maximum")) -> ()  [unwired: 2 in, 2 out]
            n122 = local write "Test Slider"(w211) -> ()
            n123 = property on="Motor" class="Clust (strict)"("Visible"=w210) -> ()  [unwired: 2 in, 2 out]
            n124 = property on="Rev/Fwd" class="Clust (strict)"("Visible"=w210) -> ()  [unwired: 2 in, 2 out]
            n125 = property on="On/Off" class="Bool (strict)"("Visible"=w210) -> ()  [unwired: 2 in, 2 out]
            n126 = property on="Test Ring" class="Ring (strict)"("Visible"=w210) -> ()  [unwired: 2 in, 2 out]
          }
          frame "Relay", "Solenoid" {
            w213 = FALSE ("Visible")
            n127 = property on="Motor" class="Clust (strict)"("Visible"=w213) -> ()  [unwired: 2 in, 2 out]
            n128 = property on="Test Slider" class="Slide (strict)"("Visible"=w213) -> ()  [unwired: 2 in, 2 out]
            n129 = Search and Replace String(input string=w214, search string="/Value  **", replace string="/Direction") -> (result string=w220:string)  [unwired: 5 in, 3 out]
            n130 = property on="Test Ring" class="Ring (strict)"("Visible"=w213) -> ()  [unwired: 2 in, 2 out]
            n131 = call <vilib>:"NT Read String.vi"("name"=w220) -> ("value"=w218:string)  [unwired: 8 in, 2 out]
            n132 = Equal?(x="Both directions", y=w218) -> (x = y?=w216:bool)
            n133 = Not(x=w216) -> (.not. x?=w217:bool)
            n134 = property on="Rev/Fwd" class="Clust (strict)"("Visible"=w216) -> ()  [unwired: 2 in, 2 out]
            n135 = property on="On/Off" class="Bool (strict)"("Visible"=w217, "Caption.Text"=w215) -> ()  [unwired: 2 in, 2 out]
          }
          frame "Compressor", "Digital Out" {
            w223 = FALSE ("Visible")
            # "Get direction and finish"
            n136 = property on="Motor" class="Clust (strict)"("Visible"=w223) -> ()  [unwired: 2 in, 2 out]
            n137 = property on="Test Slider" class="Slide (strict)"("Visible"=w223) -> ()  [unwired: 2 in, 2 out]
            n138 = property on="Test Ring" class="Ring (strict)"("Visible"=w223) -> ()  [unwired: 2 in, 2 out]
            n139 = property on="On/Off" class="Bool (strict)"("Visible"=TRUE, "Caption.Text"=w224) -> ()  [unwired: 2 in, 2 out]
            n140 = property on="Rev/Fwd" class="Clust (strict)"("Visible"=FALSE) -> ()  [unwired: 2 in, 2 out]
          }
          frame "Camera" {
            n141 = call <vilib>:"NT_Get Last Path Segment.vi"("String in"=w231) -> ("String out"=w232:string)  [unwired: 10 in]
            n142 = property on="On/Off" class="Bool (strict)"("Visible"=FALSE) -> ()  [unwired: 2 in, 2 out]
            n143 = property on="Motor" class="Clust (strict)"("Visible"=FALSE) -> ()  [unwired: 2 in, 2 out]
            n144 = property on="Rev/Fwd" class="Clust (strict)"("Visible"=FALSE) -> ()  [unwired: 2 in, 2 out]
            n145 = case shown="\"White Balance  **\"" w232 {
              tunnel: w231 -> [w238 w247 w256 w265 w274 _ w280]
              tunnel: w230 -> [w236 w244 w253 w262 w271 _ _]
              frame "Size  **" {
                n146 = Index Array(array=w236) -> (element=w235:cluster{string[]})  [unwired: 1 in]
                n147 = call <vilib>:"NT Read String.vi"("name"=w238) -> ("value"=w237:string)  [unwired: 8 in, 2 out]
                n148 = Unbundle(w235) -> (w233:string[])
                n149 = Match First String(2:w233, 3:w237) -> (0:w234:i32)  [unwired: 1 out]
                n150 = property on="Test Ring" class="Ring (strict)"("Value"=w234, "Strings []"=w233) -> ()  [unwired: 2 in, 2 out]
                n151 = property on="Test Ring" class="Ring (strict)"("Visible"=TRUE) -> ()  [unwired: 2 in, 2 out]
                n152 = property on="Test Slider" class="Slide (strict)"("Visible"=FALSE) -> ()  [unwired: 2 in, 2 out]
              }
              frame "White Balance  **" {
                n153 = Index Array(array=w244, index=1) -> (element=w245:cluster{string[]})
                n154 = call <vilib>:"NT Read String.vi"("name"=w247) -> ("value"=w246:string)  [unwired: 8 in, 2 out]
                n155 = Unbundle(w245) -> (w242:string[])
                n156 = Match First String(2:w242, 3:w246) -> (0:w241:i32)  [unwired: 1 out]
                n157 = property on="Test Ring" class="Ring (strict)"("Value"=w241, "Strings []"=w242) -> ()  [unwired: 2 in, 2 out]
                n158 = property on="Test Ring" class="Ring (strict)"("Visible"=TRUE) -> ()  [unwired: 2 in, 2 out]
                n159 = property on="Test Slider" class="Slide (strict)"("Visible"=FALSE) -> ()  [unwired: 2 in, 2 out]
              }
              frame "Exposure  **" {
                n160 = Index Array(array=w253, index=2) -> (element=w254:cluster{string[]})
                n161 = call <vilib>:"NT Read String.vi"("name"=w256) -> ("value"=w255:string)  [unwired: 8 in, 2 out]
                n162 = Unbundle(w254) -> (w250:string[])
                n163 = Match First String(2:w250, 3:w255) -> (0:w251:i32)  [unwired: 1 out]
                n164 = property on="Test Ring" class="Ring (strict)"("Value"=w251, "Strings []"=w250) -> ()  [unwired: 2 in, 2 out]
                n165 = property on="Test Ring" class="Ring (strict)"("Visible"=TRUE) -> ()  [unwired: 2 in, 2 out]
                n166 = property on="Test Slider" class="Slide (strict)"("Visible"=FALSE) -> ()  [unwired: 2 in, 2 out]
              }
              frame "Exposure Priority  **" {
                n167 = Index Array(array=w262, index=3) -> (element=w263:cluster{string[]})
                n168 = call <vilib>:"NT Read String.vi"("name"=w265) -> ("value"=w264:string)  [unwired: 8 in, 2 out]
                n169 = Unbundle(w263) -> (w259:string[])
                n170 = Match First String(2:w259, 3:w264) -> (0:w260:i32)  [unwired: 1 out]
                n171 = property on="Test Ring" class="Ring (strict)"("Value"=w260, "Strings []"=w259) -> ()  [unwired: 2 in, 2 out]
                n172 = property on="Test Ring" class="Ring (strict)"("Visible"=TRUE) -> ()  [unwired: 2 in, 2 out]
                n173 = property on="Test Slider" class="Slide (strict)"("Visible"=FALSE) -> ()  [unwired: 2 in, 2 out]
              }
              frame "Color Enable  **" {
                n174 = Index Array(array=w271, index=4) -> (element=w272:cluster{string[]})
                n175 = call <vilib>:"NT Read String.vi"("name"=w274) -> ("value"=w273:string)  [unwired: 8 in, 2 out]
                n176 = Unbundle(w272) -> (w268:string[])
                n177 = Match First String(2:w268, 3:w273) -> (0:w269:i32)  [unwired: 1 out]
                n178 = property on="Test Ring" class="Ring (strict)"("Value"=w269, "Strings []"=w268) -> ()  [unwired: 2 in, 2 out]
                n179 = property on="Test Ring" class="Ring (strict)"("Visible"=TRUE) -> ()  [unwired: 2 in, 2 out]
                n180 = property on="Test Slider" class="Slide (strict)"("Visible"=FALSE) -> ()  [unwired: 2 in, 2 out]
              }
              frame Default {
                n181 = property on="Test Ring" class="Ring (strict)"("Visible"=FALSE) -> ()  [unwired: 2 in, 2 out]
                n182 = property on="Test Slider" class="Slide (strict)"("Visible"=FALSE) -> ()  [unwired: 2 in, 2 out]
              }
              frame "Brightness  **", "Color Level  **", "Compression  **", "FPS  **", "Sharpness  **" {
                n183 = call <vilib>:"NT Read Number.vi"("name"=w280) -> ("value"=w279:dbl)  [unwired: 8 in, 2 out]
                n184 = local write "Test Slider"(w279) -> ()
                n185 = property on="Test Slider" class="Slide (strict)"("Visible"=TRUE, "Scale.Maximum"=100.0 ("Scale.Range:Maximum")) -> ()  [unwired: 2 in, 2 out]
                n186 = property on="Test Ring" class="Ring (strict)"("Visible"=FALSE) -> ()  [unwired: 2 in, 2 out]
              }
            }
          }
        }
        n187 = property on="Progress" class="Clust (strict)"("Visible"=FALSE) -> ()  [unwired: 2 in, 2 out]
      }
      event "Test Name": Mouse Enter {
        # "Populate the ring with the list of tests"
        n188 = event-data() -> ()  [unwired: 1 in, 1 out]
        n189 = call <vilib>:"NT Read String Array.vi"("name"="TestMode/TestList" ("Name")) -> ("value"=w287:string[])  [unwired: 8 in, 2 out]
        n190 = Build Array (concatenate)("Select the test to run...", w287) -> (w286:string[])
        n191 = property on="Test Name" class="Ring (strict)"("Strings []"=w286) -> ()  [unwired: 2 in, 2 out]
      }
      event "Test Name": Value Change {
        w288 = FALSE ("Visible")
        # "Tell the robot the test name to run"
        n192 = event-data() -> ("NewVal"=w292:u16)  [unwired: 1 in]
        n193 = property on="Test Name" class="Ring (strict)"() -> ("Strings []"=w293:string[])  [unwired: 2 in, 2 out]
        n194 = local write "Progress"(T5 {"Test Progress"=0, "Test Progress Text"=""} ("Progress")) -> ()
        n195 = Index Array(array=w293, index=w292) -> (element=w291:string)
        n196 = call <vilib>:"NT Write String.vi"("value"=w291, "name"="TestMode/TestName" ("Name")) -> ()  [unwired: 9 in, 1 out]
        n197 = property on="Progress" class="Clust (strict)"("Visible"=TRUE) -> ()  [unwired: 2 in, 2 out]
        n198 = property on="Motor" class="Clust (strict)"("Visible"=w288) -> ()  [unwired: 2 in, 2 out]
        n199 = property on="Test Slider" class="Slide (strict)"("Visible"=w288) -> ()  [unwired: 2 in, 2 out]
        n200 = property on="On/Off" class="Bool (strict)"("Visible"=w288) -> ()  [unwired: 2 in, 2 out]
        n201 = property on="Rev/Fwd" class="Clust (strict)"("Visible"=w288) -> ()  [unwired: 2 in, 2 out]
        n202 = property on="Test Ring" class="Ring (strict)"("Visible"=w288) -> ()  [unwired: 2 in, 2 out]
      }
      event "Select Auto": Mouse Enter {
        # "Populate the combo box with the list of autonomous options"
        n203 = event-data() -> ()  [unwired: 1 in, 1 out]
        n204 = call <vilib>:"NT Read String Array.vi"("name"="Auto List" ("Name")) -> ("value"=w295:string[])  [unwired: 8 in, 2 out]
        n205 = property on="Select Auto" class="CmbBox"("Strings[]"=w295) -> ()  [unwired: 2 in, 2 out]
      }
      event "Select Auto": Value Change {
        # "User modified the Auto Selection. Write to NT variable so robot knows."
        n206 = event-data() -> ("NewVal"=w297:string)  [unwired: 1 in]
        n207 = call <vilib>:"NT Write String.vi"("value"=w297, "name"="Auto Selector" ("Name")) -> ()  [unwired: 9 in, 1 out]
      }
      event "CheckList": Double Click {
        # "Shift clears all"
        # "Update symbols on the listbox"
        n208 = event-data() -> ("PlatMods.Shift"=w299:bool, "Row"=w301:i32)  [unwired: 1 in]
        n209 = case shown="True" w299 {
          tunnel: w301 -> [w305 _]
          tunnel: 1 -> [w304 _]
          frame False {
            n210 = property on="CheckList" class="LstBox (strict)"() -> ("Item Symbols"=w303:i32[])  [unwired: 2 in, 2 out]
            n211 = Replace Array Subset(array=w303, new element=w304, index=w305) -> (w302:i32[])
            n212 = property on="CheckList" class="LstBox (strict)"("Item Symbols"=w302) -> ()  [unwired: 2 in, 2 out]
          }
          frame True {
            w306 = 0 ("Top Row")
            n213 = property on="CheckList" class="LstBox (strict)"() -> ("Number of Rows"=w308:u32)  [unwired: 2 in, 2 out]
            n214 = Initialize Array(0, w308) -> (w307:i32[])
            n215 = property on="CheckList" class="LstBox (strict)"("Top Row"=w306, "Value"=w306, "Item Symbols"=w307) -> ()  [unwired: 2 in, 2 out]
          }
        }
      }
      event "CheckList": Key Down {
        # "Update symbols on the listbox\nLeft and right keys check and uncheck"
        n216 = event-data() -> ("VKey"=w311:T22)  [unwired: 1 in]
        n217 = case shown="\"Left\", \"Right\"" w311 {
          selector: w311 -> [w316 _]
          tunnel: eventvkey."Left" ("VKey") -> [w314 _]
          frame "Left", "Right" {
            n218 = Equal?(x=w314, y=w316) -> (x = y?=w315:bool)
            n219 = Select(t=0, s=w315, f=1) -> (s? t:f=w317:i32)
            n220 = property on="CheckList" class="LstBox (strict)"() -> ("Item Symbols"=w320:i32[])  [unwired: 2 in, 2 out]
            n221 = Replace Array Subset(array=w320, new element=w317, index="CheckList") -> (w319:i32[])
            n222 = property on="CheckList" class="LstBox (strict)"("Item Symbols"=w319) -> ()  [unwired: 2 in, 2 out]
          }
          frame Default {
          }
        }
      }
      event "Motor.Enable": Value Change {
        # "When the test mode otor enable helper is set, update that\ntree row item's value"
        n223 = event-data() -> ("NewVal"=w325:bool)  [unwired: 1 in]
        n224 = Unbundle("Motor") -> ("Value"=w324:dbl)  [unwired: 1 out]
        n225 = Select(t=w324, s=w325, f=0.0) -> (s? t:f=w322:dbl)
        n226 = call <vilib>:"NT Write Number.vi"("value"=w322, "name"=w321) -> ()  [unwired: 9 in, 1 out]
      }
      event "Test Slider": Value Change {
        # "When the test mode slider helper is set, update that\ntree row item's value"
        n227 = event-data() -> ("NewVal"=w327:dbl)  [unwired: 1 in]
        n228 = call <vilib>:"NT Write Number.vi"("value"=w327, "name"=w328) -> ()  [unwired: 9 in, 1 out]
      }
      event "On/Off": Value Change {
        # "When the test mode on/off helper value is set, update that\ntree row item's value"
        n229 = event-data() -> ("NewVal"=w331:bool)  [unwired: 1 in]
        n230 = Boolean To (0,1)(Boolean=w331) -> (0, 1=w330:i16)
        n231 = call <vilib>:"NT Write Number.vi"("value"=w330, "name"=w329) -> ()  [unwired: 9 in, 1 out]
      }
      event "Rev/Fwd": Value Change {
        # "When the test mode helper value for relays is set, update that\ntree row item's value"
        n232 = event-data() -> ("NewVal.Forward"=w338:bool, "NewVal.Reverse"=w337:bool)  [unwired: 1 in]
        n233 = Boolean To (0,1)(Boolean=w338) -> (0, 1=w334:i16)
        n234 = Boolean To (0,1)(Boolean=w337) -> (0, 1=w336:i16)
        n235 = Negate(x=w336) -> (-x=w335:i16)
        n236 = Add(x=w334, y=w335) -> (x+y=w333:i16)
        n237 = call <vilib>:"NT Write Number.vi"("value"=w333, "name"=w332) -> ()  [unwired: 9 in, 1 out]
      }
      event "Test Ring": Value Change {
        # "When a test mode helper value is selected from the ring,\nset the tree item's variable to the string value"
        n238 = event-data() -> ("NewVal"=w341:u16)  [unwired: 1 in]
        n239 = property on="Test Ring" class="Ring (strict)"() -> ("Strings []"=w342:string[])  [unwired: 2 in, 2 out]
        n240 = Index Array(array=w342, index=w341) -> (element=w340:string)
        n241 = call <vilib>:"NT Write String.vi"("value"=w340, "name"=w339) -> ()  [unwired: 9 in, 1 out]
      }
      event "Rec Mode": Value Change {
        # "Update globals for recording mode and path to read log from.\nClear when logging and let NetworkTables set path for vision to\nuse."
        n242 = event-data() -> ("NewVal"=w351:enum32{"Stop", "Record", "Playback"})  [unwired: 1 in]
        n243 = global write "WPI_DashboardLogging Global.vi" "Logging Filename"(path "") -> ()
        n244 = global write "WPI_DashboardLogging Global.vi" "Recording"(w351) -> ()
        n245 = case shown="\"Playback\"" w351 {
          tunnel: w350 -> [_ w353 w361]
          tunnel: [_ _ w360] -> w348
          tunnel: [_ _ w359] -> _
          tunnel: w346 -> [_ _ w357]
          tunnel: cluster{i32, i32} {-250, 170} -> [_ _ w356]
          tunnel: [_ _ T23 {"Image Size"=TRUE, "Image Type"=TRUE, "Pixel Value"=TRUE, "ROI Information"=TRUE, "Zoom Factor"=FALSE} ("Image Information Shown:All Elements")] -> w343
          tunnel: [_ _ TRUE ("Zoom Factor")] -> w344
          frame Default {
          }
          frame "Stop", "Record" {
            # "Place Window too"
            n246 = invoke class="VI" method="FP.Close"(reference=w353) -> (reference out=w352:refnum<vi>)  [unwired: 2 in, 2 out]
            n247 = invoke class="VI" method="Abort VI"(reference=w352) -> ()  [unwired: 2 in, 3 out]
          }
          frame "Playback" {
            n248 = call "Open Playback Panel.vi"("Offset"=w356, "DB VI Ref"=w357, "Playback in"=w361) -> ("Playback out"=w358:refnum<vi>)  [unwired: 8 in]
            n249 = register-events(w358) -> (reference out=w360:refnum<event-registration>, error out=w359:errorcluster)  [unwired: 2 in]
          }
        }
        n250 = property on="Camera Image" class="ImageControl"("Image Information Shown"=w343, "Image Information Visible"=w344) -> ()  [unwired: 2 in, 2 out]
        n251 = call <vilib>:"WPI_DashboardNT Log FieldName Cache.vi"("Operation"=enum16{"Lookup/Add", "Index", "Clear"}."Clear") -> ()  [unwired: 8 in, 3 out]
      }
      event Panel Close {
        w362 = enum32{"Stop", "Record", "Playback"}."Stop" ("Rec Mode")
        # "Playback window has been closed, abort"
        n252 = event-data() -> ()  [unwired: 1 in, 4 out]
        n253 = local write "Rec Mode"(w362) -> ()
        n254 = global write "WPI_DashboardLogging Global.vi" "Recording"(w362) -> ()
      }
      event Panel Close {
        # "Abort playback window and ourself"
        n255 = event-data() -> ()  [unwired: 1 in, 4 out]
        n256 = invoke class="VI" method="FP.Close"(reference=w365) -> (reference out=w364:refnum<vi>)  [unwired: 2 in, 2 out]
        n257 = invoke class="VI" method="Abort VI"(reference=w364) -> (error out=w363:errorcluster)  [unwired: 2 in, 2 out]
        n258 = invoke class="VI" method="Abort VI"(error in=w363) -> ()  [unwired: 2 in, 3 out]
      }
      event "Tree": Double Click {
        n259 = event-data() -> ("PlatMods"=w371:T25, "Tag"=w368:string)  [unwired: 1 in]
        n260 = Unbundle(w371) -> ("Shift"=w370:bool)  [unwired: 4 out]
        n261 = String Subset(string=w368, length (rest)=1 ("length (rest)")) -> (substring=w367:string)  [unwired: 1 in]
        n262 = Not(x=w370) -> (.not. x?=w369:bool)
        n263 = case shown="\"/\"" w367 {
          tunnel: w368 -> [_ w373]
          tunnel: w369 -> [_ w372]
          frame Default {
          }
          frame "/" {
            n264 = call <vilib>:"NT Update Persistence.vi"("Persistence"=w372, "Name"=w373) -> ()  [unwired: 9 in, 1 out]
          }
        }
      }
    }
  }
  n265 = while {
    tunnel: w44 -> [w375]
    i -> [w378]
    stop <- FALSE stop-if-true
    n266 = Wait (ms)(milliseconds to wait=u32 100) -> ()  [unwired: 1 out]
    n267 = case shown="\"Playback\"" "Rec Mode" {
      tunnel: w378 -> [_ _ w393]
      tunnel: [u32 2829099 ("Base Color") u32 11141120 ("Target Color") w382] -> w374
      frame "Stop", Default {
        # "Reset the color, extra updates don't cost much"
      }
      frame "Record" {
      }
      frame "Playback" {
        # "Playback"
        n268 = Quotient & Remainder(x=w393, y=u32 50 ("milliseconds to wait")) -> (x-y*floor(x/y)=w389:u32)  [unwired: 1 out]
        n269 = Divide(x=w389, y=u32 50 ("milliseconds to wait")) -> (x/y=w386:dbl)
        n270 = Multiply(x=6.283185307179586, y=w386) -> (x*y=w391:dbl)
        n271 = Sine(x=w391) -> (sin(x)=w390:dbl)
        n272 = Absolute Value(x=w390) -> (abs(x)=w383:dbl)
        n273 = call "Interpolate RGB Color.vi"("Proportion"=w383, "Target Color"=u32 30976, "Base Color"=u32 2829099) -> ("Result Color"=w382:u32)  [unwired: 8 in]
      }
    }
    n274 = property class="Pane"(reference=w375, "PaneColor"=w374) -> ()  [unwired: 1 in, 2 out]
  }
  n275 = local write "Dashboard Tab"(T7."Drive" ("Dashboard Tab")) -> ()
  n276 = property on="On/Off" class="Bool (strict)"("Visible"=w17) -> ()  [unwired: 2 in, 2 out]
  n277 = property on="Motor" class="Clust (strict)"("Visible"=w17) -> ()  [unwired: 2 in, 2 out]
  n278 = property on="Progress" class="Clust (strict)"("Visible"=w17) -> ()  [unwired: 2 in, 2 out]
  n279 = property on="Test Ring" class="Ring (strict)"("Visible"=w17) -> ()  [unwired: 2 in, 2 out]
  n280 = property on="Rev/Fwd" class="Clust (strict)"("Visible"=w17) -> ()  [unwired: 2 in, 2 out]
  n281 = while {
    tunnel: u16 1741 ("timeout ms (25000)") -> [w395]
    stop <- FALSE stop-if-true
    n282 = TCP Create Listener(10:w395) -> (0:w394:errorcluster, 3:w396:refnum<k5>)  [unwired: 4 in, 1 out]
    n283 = case shown="No Error" w394 {
      selector: w394 -> [w398 _]
      tunnel: w396 -> [w399 _]
      frame No Error {
        n284 = while {
          tunnel: w399 -> [w402]
          tunnel: w398 -> [w401]
          stop <- FALSE stop-if-true
          n285 = TCP Wait On Listener(8:w401, 11:w402) -> (0:w403:errorcluster, 4:w404:refnum<k5>)  [unwired: 2 in, 3 out]
          n286 = local write "TCP"(w404) -> ()
          n287 = case shown="Error" w403 {
            frame No Error {
            }
            frame Error {
              n288 = Wait (ms)(milliseconds to wait=u32 1000) -> ()  [unwired: 1 out]
            }
          }
        }
      }
      frame Error {
        n289 = Wait (ms)(milliseconds to wait=u32 1000) -> ()  [unwired: 1 out]
      }
    }
  }
  n290 = global write "WPI_DashboardLogging Global.vi" "Recording"(w39) -> ()
  n291 = local write "Rec Mode"(w39) -> ()
  n292 = call <vilib>:"NT Write String.vi"("value"="Select Auto", "name"="Auto Selector" ("Name")) -> ()  [unwired: 9 in, 1 out]
